vi "HW_set_IO_ports_3-pos_2.vi"(0 "IO parameters cluster":T1) -> (1 "IO parameters cluster output":T1, 2 "IO changed":bool)   [LabVIEW 2018, in "Tracker.lvlib"]
uses:
  Tracker.lvlib
  Controls/CTL_IO_params_cluster.ctl
  <vilib>/Utility/miscctls.llb/LVPointTypeDef.ctl
panel:
  out "In tag":string
  out "Out tag":string
  in  "IO 4 invert":bool caption="Swap High/Low"
  in  "IO 3 invert":bool caption="Swap High/Low"
  in  "IO 2 invert":bool caption="Swap High/Low"
  in  "IO 1 invert":bool caption="Swap High/Low"
  in  "IO 4":u16(ring)=1 items=["Out", "In"]
  in  "IO 3":u16(ring)=1 items=["Out", "In"]
  in  "IO 2":u16(ring) items=["Out", "In", "Sync (p)"]
  in  "IO 1":u16(ring) items=["Out", "In", "Sync (t)"]
  in  "Activate ext. RS-232":bool
  in  "Reset IO":bool
  in  "IO 4 start/stop":bool caption="Send TTL at Start and Stop"
  in  "IO 3 start/stop":bool caption="Send TTL at Start and Stop"
  in  "IO 2 start/stop":bool caption="Initiate outgoing TTL pulse"
  in  "IO 1 start/stop":bool caption="Initiate outgoing TTL pulse"
  in  "Exit":bool
  in  "Save Settings":bool
  in  "IO 4 zone":bool
  in  "IO 3 zone":bool
  in  "IO 2 sync":bool
  in  "IO 2 zone":bool=TRUE
  in  "IO 1 sync":bool
  in  "IO 1 zone":bool=TRUE
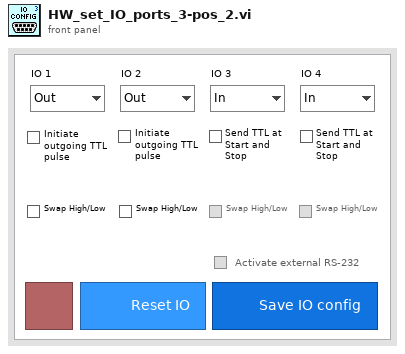
[diagram p1: front panel]
types:
  T1 = typedef "Tracker.lvlib/CTL_IO_params_cluster.ctl" = cluster{"IO general config.":u16, "IO 1 configuration":u16, "IO 2 configuration":u16, "IO 3 configuration":u16, "IO 4 configuration":u16, "Activate ext. RS-232":u16, "IO inversion config.":u16, "Sync capability":u8}
  T2 = typedef "LVPointTypeDef.ctl" = cluster{"Horizontal":i16, "Vertical":i16}
  T3 = enum8{"Enabled", "Disabled", "Disabled and Grayed Out"}
  T4 = cluster{"IO general config.":bool, "IO 1 configuration":bool, "IO 2 configuration":bool, "IO 3 configuration":bool, "IO 4 configuration":bool, "Activate ext. RS-232":bool, "IO inversion config.":bool, "Sync capability":bool}
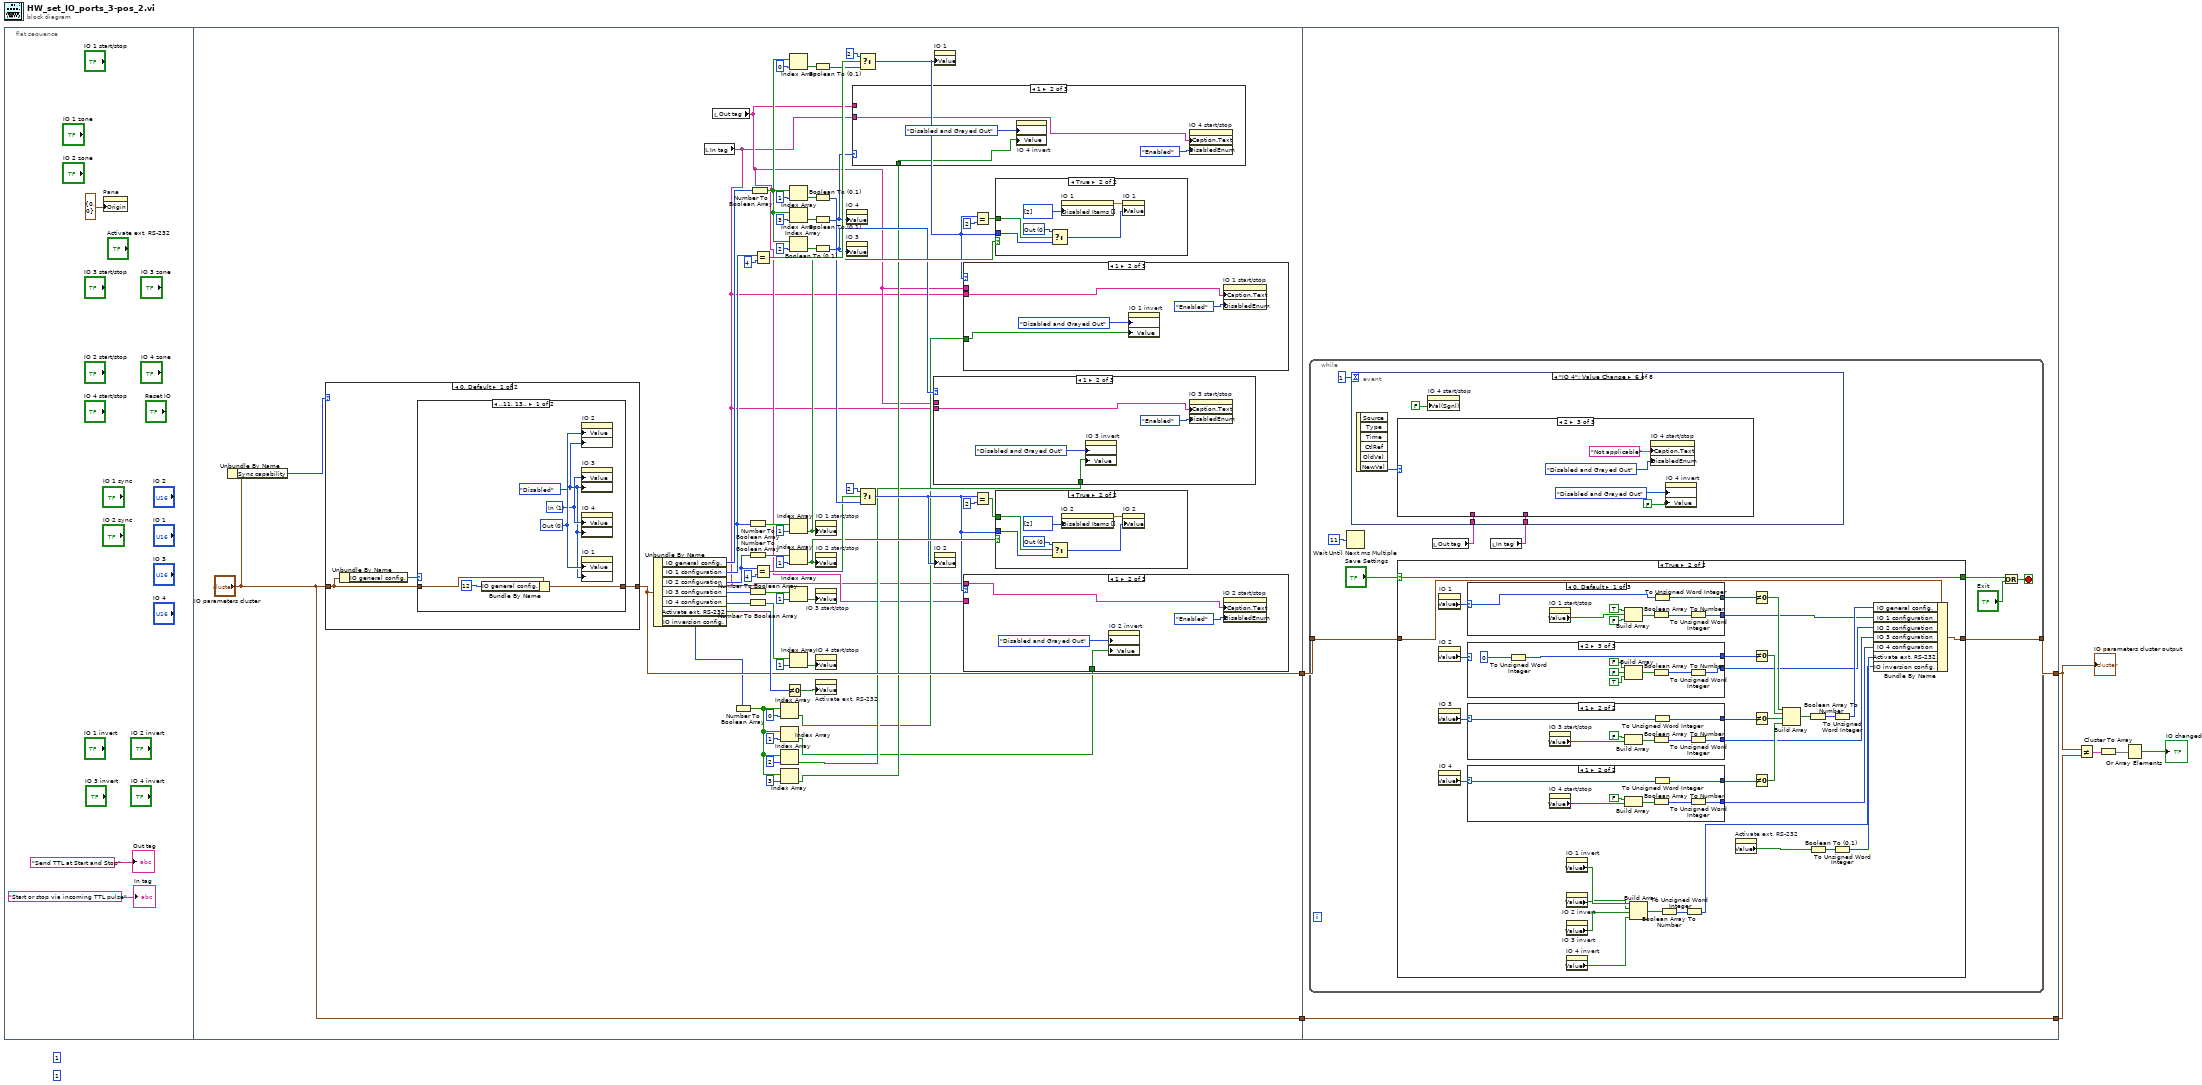
[diagram p0: block diagram]
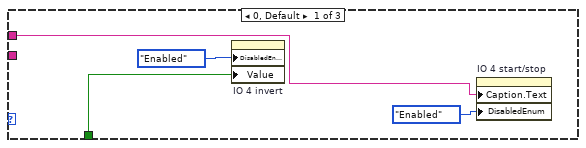
[diagram p2: hidden frame]
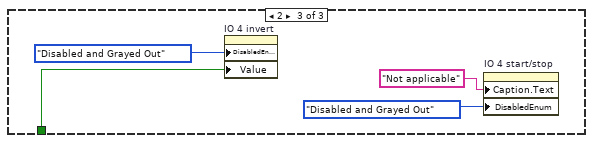
[diagram p3: hidden frame]
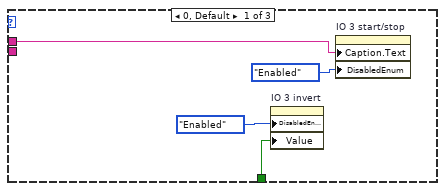
[diagram p4: hidden frame]
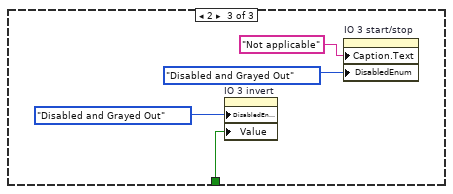
[diagram p5: hidden frame]
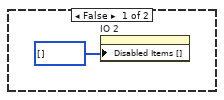
[diagram p6: hidden frame]
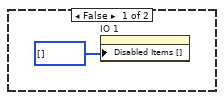
[diagram p7: hidden frame]
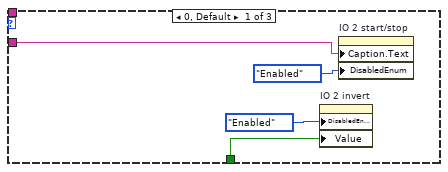
[diagram p8: hidden frame]
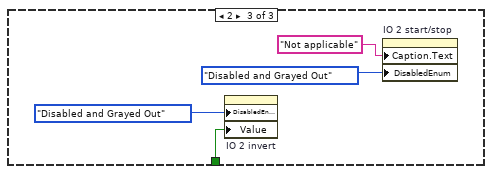
[diagram p9: hidden frame]
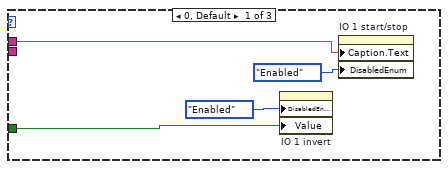
[diagram p10: hidden frame]
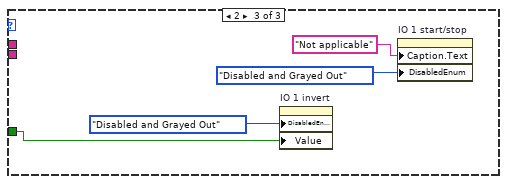
[diagram p11: hidden frame]
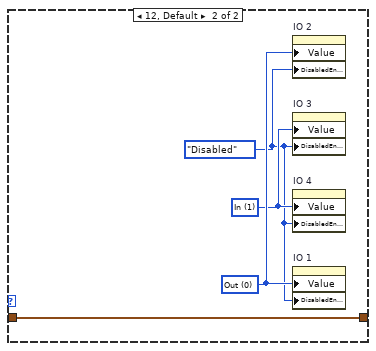
[diagram p12: hidden frame]
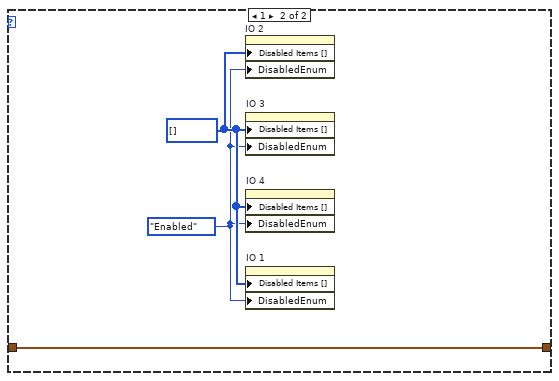
[diagram p13: hidden frame]
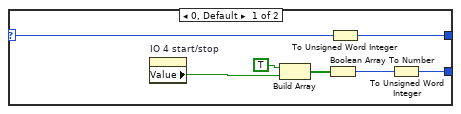
[diagram p15: hidden frame]
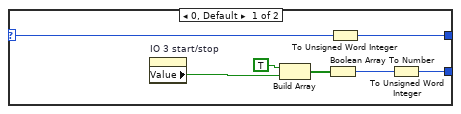
[diagram p16: hidden frame]
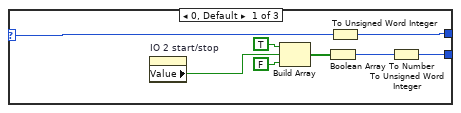
[diagram p17: hidden frame]
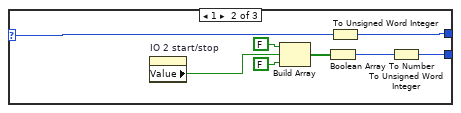
[diagram p18: hidden frame]
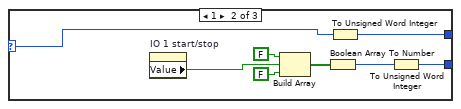
[diagram p19: hidden frame]
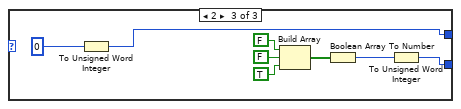
[diagram p20: hidden frame]
diagram:
  (unwired) 1 ("index")
  (unwired) 1 ("index")
  n1 = flat-sequence {
    tunnel: [w49] -> w7
    tunnel: ["IO parameters cluster"] -> w6
    tunnel: [w150] -> w5
    tunnel: w7 -> [w149]
    tunnel: w6 -> [w148]
    tunnel: [w148] -> w4
    frame #0 {
      n2 = property on="Pane" class="Pane"("Origin"=T2 {"Horizontal"=0, "Vertical"=0}) -> ()  [unwired: 2 in, 2 out]
      "In tag" <- "Start or stop via incoming TTL pulse" ("In tag")
      "Out tag" <- "Send TTL at Start and Stop" ("Out tag")
    }
    frame #1 {
      n3 = Unbundle By Name("IO parameters cluster") -> ("Sync capability"=w14:u8)
      n4 = case shown="0, Default" w14 {
        tunnel: "IO parameters cluster" -> [w133 w147]
        tunnel: [w132 w147] -> w49
        frame 0, Default {
          n5 = Unbundle By Name(w133) -> ("IO general config."=w134:u16)
          n6 = case shown="..11, 13.." w134 {
            tunnel: [w139 w144] -> w132
            tunnel: w133 -> [w140 w144]
            frame ..11, 13.. {
              w135 = T3."Disabled" ("Disabled")
              w136 = u16 1 items=["Out", "In"] ("IO 3")
              w137 = u16 0 items=["Out", "In", "Sync (t)"] ("IO 1")
              n7 = Bundle By Name(cluster=w140, "IO general config."=u16 12 ("SYNC configuration")) -> (w139:T1)
              n8 = property on="IO 2" class="Ring (strict)"("Value"=w137, "DisabledEnum"=w135) -> ()  [unwired: 2 in, 2 out]
              n9 = property on="IO 3" class="Ring (strict)"("Value"=w136, "DisabledEnum"=w135) -> ()  [unwired: 2 in, 2 out]
              n10 = property on="IO 4" class="Ring (strict)"("Value"=w136, "DisabledEnum"=w135) -> ()  [unwired: 2 in, 2 out]
              n11 = property on="IO 1" class="Ring (strict)"("Value"=w137, "DisabledEnum"=w135) -> ()  [unwired: 2 in, 2 out]
            }
            frame 12, Default {
              w141 = T3."Disabled" ("Disabled")
              w142 = u16 1 items=["Out", "In"] ("IO 3")
              w143 = u16 0 items=["Out", "In", "Sync (t)"] ("IO 1")
              n12 = property on="IO 2" class="Ring (strict)"("Value"=w143, "DisabledEnum"=w141) -> ()  [unwired: 2 in, 2 out]
              n13 = property on="IO 3" class="Ring (strict)"("Value"=w142, "DisabledEnum"=w141) -> ()  [unwired: 2 in, 2 out]
              n14 = property on="IO 4" class="Ring (strict)"("Value"=w142, "DisabledEnum"=w141) -> ()  [unwired: 2 in, 2 out]
              n15 = property on="IO 1" class="Ring (strict)"("Value"=w143, "DisabledEnum"=w141) -> ()  [unwired: 2 in, 2 out]
            }
          }
        }
        frame 1 {
          w145 = T3."Enabled" ("Disabled")
          w146 = i32[] [] ("Disabled Items []")
          n16 = property on="IO 2" class="Ring (strict)"("Disabled Items []"=w146, "DisabledEnum"=w145) -> ()  [unwired: 2 in, 2 out]
          n17 = property on="IO 3" class="Ring (strict)"("Disabled Items []"=w146, "DisabledEnum"=w145) -> ()  [unwired: 2 in, 2 out]
          n18 = property on="IO 4" class="Ring (strict)"("Disabled Items []"=w146, "DisabledEnum"=w145) -> ()  [unwired: 2 in, 2 out]
          n19 = property on="IO 1" class="Ring (strict)"("Disabled Items []"=w146, "DisabledEnum"=w145) -> ()  [unwired: 2 in, 2 out]
        }
      }
      n20 = Unbundle By Name(w49) -> ("IO general config."=w69:u16, "IO 1 configuration"=w44:u16, "IO 2 configuration"=w36:u16, "IO 3 configuration"=w53:u16, "IO 4 configuration"=w52:u16, "Activate ext. RS-232"=w51:u16, "IO inversion config."=w24:u16)
      n21 = local read "In tag"() -> (w11:string)
      n22 = local read "Out tag"() -> (w12:string)
      n23 = Number To Boolean Array(number=w24) -> (Boolean array=w19:bool[])
      n24 = Number To Boolean Array(number=w44) -> (Boolean array=w59:bool[])
      n25 = Number To Boolean Array(number=w36) -> (Boolean array=w56:bool[])
      n26 = Number To Boolean Array(number=w53) -> (Boolean array=w55:bool[])
      n27 = Number To Boolean Array(number=w52) -> (Boolean array=w45:bool[])
      n28 = Number To Boolean Array(number=w69) -> (Boolean array=w68:bool[])
      n29 = Equal?(x=w44, y=u16 4) -> (x = y?=w42:bool)
      n30 = Equal?(x=w36, y=u16 4) -> (x = y?=w35:bool)
      n31 = Index Array(array=w19, index=0) -> (element=w15:bool)
      n32 = Index Array(array=w19, index=1) -> (element=w16:bool)
      n33 = Index Array(array=w19, index=2) -> (element=w17:bool)
      n34 = Index Array(array=w19, index=3) -> (element=w18:bool)
      n35 = Not Equal To 0?(x=w51) -> (x != 0?=w50:bool)
      n36 = Index Array(array=w68, index=0) -> (element=w63:bool)
      n37 = Index Array(array=w68, index=1) -> (element=w62:bool)
      n38 = Index Array(array=w68, index=3) -> (element=w60:bool)
      n39 = Index Array(array=w68, index=2) -> (element=w61:bool)
      n40 = Index Array(array=w59, index=1) -> (element=w33:bool)
      n41 = Index Array(array=w56, index=1) -> (element=w28:bool)
      n42 = Index Array(array=w55, index=1) -> (element=w54:bool)
      n43 = Index Array(array=w45, index=1) -> (element=w46:bool)
      n44 = Boolean To (0,1)(Boolean=w63) -> (0, 1=w41:i16)
      n45 = Boolean To (0,1)(Boolean=w62) -> (0, 1=w38:i16)
      n46 = Boolean To (0,1)(Boolean=w60) -> (0, 1=w25:i16)
      n47 = Boolean To (0,1)(Boolean=w61) -> (0, 1=w26:i16)
      n48 = property on="IO 1 start/stop" class="Bool (strict)"("Value"=w33) -> ()  [unwired: 2 in, 2 out]
      n49 = property on="IO 2 start/stop" class="Bool (strict)"("Value"=w28) -> ()  [unwired: 2 in, 2 out]
      n50 = property on="IO 3 start/stop" class="Bool (strict)"("Value"=w54) -> ()  [unwired: 2 in, 2 out]
      n51 = property on="IO 4 start/stop" class="Bool (strict)"("Value"=w46) -> ()  [unwired: 2 in, 2 out]
      n52 = property on="Activate ext. RS-232" class="Bool (strict)"("Value"=w50) -> ()  [unwired: 2 in, 2 out]
      n53 = property on="IO 4" class="Ring (strict)"("Value"=w25) -> ()  [unwired: 2 in, 2 out]
      n54 = property on="IO 3" class="Ring (strict)"("Value"=w26) -> ()  [unwired: 2 in, 2 out]
      n55 = case shown="1" w25 {
        tunnel: w18 -> [w71 w75 w78]
        tunnel: w12 -> [w70 _ _]
        tunnel: w11 -> [_ w74 _]
        frame 0, Default {
          n56 = property on="IO 4 invert" class="Bool (strict)"("DisabledEnum"=T3."Enabled" ("Disabled"), "Value"=w71) -> ()  [unwired: 2 in, 2 out]
          n57 = property on="IO 4 start/stop" class="Bool (strict)"("Caption.Text"=w70, "DisabledEnum"=T3."Enabled" ("Disabled")) -> ()  [unwired: 2 in, 2 out]
        }
        frame 1 {
          n58 = property on="IO 4 invert" class="Bool (strict)"("DisabledEnum"=T3."Disabled and Grayed Out" ("Disabled"), "Value"=w75) -> ()  [unwired: 2 in, 2 out]
          n59 = property on="IO 4 start/stop" class="Bool (strict)"("Caption.Text"=w74, "DisabledEnum"=T3."Enabled" ("Disabled")) -> ()  [unwired: 2 in, 2 out]
        }
        frame 2 {
          n60 = property on="IO 4 invert" class="Bool (strict)"("DisabledEnum"=T3."Disabled and Grayed Out" ("Disabled"), "Value"=w78) -> ()  [unwired: 2 in, 2 out]
          n61 = property on="IO 4 start/stop" class="Bool (strict)"("Caption.Text"="Not applicable", "DisabledEnum"=T3."Disabled and Grayed Out" ("Disabled")) -> ()  [unwired: 2 in, 2 out]
        }
      }
      n62 = Select(t=i16 2, s=w42, f=w41) -> (s? t:f=w31:i16)
      n63 = Select(t=i16 2, s=w35, f=w38) -> (s? t:f=w27:i16)
      n64 = case shown="1" w26 {
        tunnel: w17 -> [w83 w87 w90]
        tunnel: w12 -> [w82 _ _]
        tunnel: w11 -> [_ w86 _]
        frame 0, Default {
          n65 = property on="IO 3 invert" class="Bool (strict)"("DisabledEnum"=T3."Enabled" ("Disabled"), "Value"=w83) -> ()  [unwired: 2 in, 2 out]
          n66 = property on="IO 3 start/stop" class="Bool (strict)"("Caption.Text"=w82, "DisabledEnum"=T3."Enabled" ("Disabled")) -> ()  [unwired: 2 in, 2 out]
        }
        frame 1 {
          n67 = property on="IO 3 invert" class="Bool (strict)"("DisabledEnum"=T3."Disabled and Grayed Out" ("Disabled"), "Value"=w87) -> ()  [unwired: 2 in, 2 out]
          n68 = property on="IO 3 start/stop" class="Bool (strict)"("Caption.Text"=w86, "DisabledEnum"=T3."Enabled" ("Disabled")) -> ()  [unwired: 2 in, 2 out]
        }
        frame 2 {
          n69 = property on="IO 3 invert" class="Bool (strict)"("DisabledEnum"=T3."Disabled and Grayed Out" ("Disabled"), "Value"=w90) -> ()  [unwired: 2 in, 2 out]
          n70 = property on="IO 3 start/stop" class="Bool (strict)"("Caption.Text"="Not applicable", "DisabledEnum"=T3."Disabled and Grayed Out" ("Disabled")) -> ()  [unwired: 2 in, 2 out]
        }
      }
      n71 = property on="IO 1" class="Ring (strict)"("Value"=w31) -> ()  [unwired: 2 in, 2 out]
      n72 = property on="IO 2" class="Ring (strict)"("Value"=w27) -> ()  [unwired: 2 in, 2 out]
      n73 = case shown="1" w31 {
        tunnel: w15 -> [w121 w125 w128]
        tunnel: w12 -> [w120 _ _]
        tunnel: w11 -> [_ w124 _]
        frame 0, Default {
          n74 = property on="IO 1 invert" class="Bool (strict)"("DisabledEnum"=T3."Enabled" ("Disabled"), "Value"=w121) -> ()  [unwired: 2 in, 2 out]
          n75 = property on="IO 1 start/stop" class="Bool (strict)"("Caption.Text"=w120, "DisabledEnum"=T3."Enabled" ("Disabled")) -> ()  [unwired: 2 in, 2 out]
        }
        frame 1 {
          n76 = property on="IO 1 invert" class="Bool (strict)"("DisabledEnum"=T3."Disabled and Grayed Out" ("Disabled"), "Value"=w125) -> ()  [unwired: 2 in, 2 out]
          n77 = property on="IO 1 start/stop" class="Bool (strict)"("Caption.Text"=w124, "DisabledEnum"=T3."Enabled" ("Disabled")) -> ()  [unwired: 2 in, 2 out]
        }
        frame 2 {
          n78 = property on="IO 1 invert" class="Bool (strict)"("DisabledEnum"=T3."Disabled and Grayed Out" ("Disabled"), "Value"=w128) -> ()  [unwired: 2 in, 2 out]
          n79 = property on="IO 1 start/stop" class="Bool (strict)"("Caption.Text"="Not applicable", "DisabledEnum"=T3."Disabled and Grayed Out" ("Disabled")) -> ()  [unwired: 2 in, 2 out]
        }
      }
      n80 = case shown="1" w27 {
        tunnel: w16 -> [w109 w113 w116]
        tunnel: w12 -> [w108 _ _]
        tunnel: w11 -> [_ w112 _]
        frame 0, Default {
          n81 = property on="IO 2 invert" class="Bool (strict)"("DisabledEnum"=T3."Enabled" ("Disabled"), "Value"=w109) -> ()  [unwired: 2 in, 2 out]
          n82 = property on="IO 2 start/stop" class="Bool (strict)"("Caption.Text"=w108, "DisabledEnum"=T3."Enabled" ("Disabled")) -> ()  [unwired: 2 in, 2 out]
        }
        frame 1 {
          n83 = property on="IO 2 invert" class="Bool (strict)"("DisabledEnum"=T3."Disabled and Grayed Out" ("Disabled"), "Value"=w113) -> ()  [unwired: 2 in, 2 out]
          n84 = property on="IO 2 start/stop" class="Bool (strict)"("Caption.Text"=w112, "DisabledEnum"=T3."Enabled" ("Disabled")) -> ()  [unwired: 2 in, 2 out]
        }
        frame 2 {
          n85 = property on="IO 2 invert" class="Bool (strict)"("DisabledEnum"=T3."Disabled and Grayed Out" ("Disabled"), "Value"=w116) -> ()  [unwired: 2 in, 2 out]
          n86 = property on="IO 2 start/stop" class="Bool (strict)"("Caption.Text"="Not applicable", "DisabledEnum"=T3."Disabled and Grayed Out" ("Disabled")) -> ()  [unwired: 2 in, 2 out]
        }
      }
      n87 = Equal?(x=w31, y=u16 2) -> (x = y?=w34:bool)
      n88 = Equal?(x=w27, y=u16 2) -> (x = y?=w30:bool)
      n89 = case shown="True" w33 {
        tunnel: w34 -> [_ w105]
        tunnel: w31 -> [_ w102]
        frame False {
          n90 = property on="IO 1" class="Ring (strict)"("Disabled Items []"=i32[] []) -> ()  [unwired: 2 in, 2 out]
        }
        frame True {
          w104 = u16 0 items=["Out", "In", "Sync (t)"] ("IO 1")
          n91 = Select(t=w104, s=w105, f=w102) -> (s? t:f=w103:u16)
          n92 = property on="IO 1" class="Ring (strict)"("Disabled Items []"=i32[] [2]) -> (error out=w106:errorcluster)  [unwired: 2 in, 1 out]
          n93 = property on="IO 1" class="Ring (strict)"(error in=w106, "Value"=w103) -> ()  [unwired: 1 in, 2 out]
        }
      }
      n94 = case shown="True" w28 {
        tunnel: w30 -> [_ w98]
        tunnel: w27 -> [_ w95]
        frame False {
          n95 = property on="IO 2" class="Ring (strict)"("Disabled Items []"=i32[] []) -> ()  [unwired: 2 in, 2 out]
        }
        frame True {
          w97 = u16 0 items=["Out", "In", "Sync (t)"] ("IO 1")
          n96 = Select(t=w97, s=w98, f=w95) -> (s? t:f=w96:u16)
          n97 = property on="IO 2" class="Ring (strict)"("Disabled Items []"=i32[] [2]) -> (error out=w99:errorcluster)  [unwired: 2 in, 1 out]
          n98 = property on="IO 2" class="Ring (strict)"(error in=w99, "Value"=w96) -> ()  [unwired: 1 in, 2 out]
        }
      }
    }
    frame #2 {
      n99 = while {
        tunnel: [w154] -> w150
        tunnel: w149 -> [w153]
        stop <- w157 stop-if-true
        n100 = Wait Until Next ms Multiple(millisecond multiple=u32 11) -> ()  [unwired: 1 out]
        n101 = case shown="True" "Save Settings" {
          selector: "Save Settings" -> [w162 w194]
          tunnel: [w162 w194] -> w155
          tunnel: [w161 w189] -> w154
          tunnel: w153 -> [w161 w190]
          frame False {
          }
          frame True {
            n102 = property on="IO 1" class="Ring (strict)"() -> ("Value"=w191:u16)  [unwired: 2 in, 2 out]
            n103 = property on="IO 2" class="Ring (strict)"() -> ("Value"=w188:u16)  [unwired: 2 in, 2 out]
            n104 = property on="IO 3" class="Ring (strict)"() -> ("Value"=w187:u16)  [unwired: 2 in, 2 out]
            n105 = property on="IO 4" class="Ring (strict)"() -> ("Value"=w186:u16)  [unwired: 2 in, 2 out]
            n106 = case shown="0, Default" w191 {
              selector: w191 -> [w250 w258 _]
              tunnel: [w247 w255 w264] -> w174
              tunnel: [w249 w257 w267] -> w179
              frame 0, Default {
                n107 = property on="IO 1 start/stop" class="Bool (strict)"() -> ("Value"=w254:bool)  [unwired: 2 in, 2 out]
                n108 = Build Array(TRUE, w254, FALSE) -> (w251:bool[])
                n109 = Boolean Array To Number(Boolean array=w251) -> (number=w248:u32)
                n110 = To Unsigned Word Integer(number=w250) -> (unsigned 16bit integer=w249:u16)
                n111 = To Unsigned Word Integer(number=w248) -> (unsigned 16bit integer=w247:u16)
              }
              frame 1 {
                n112 = property on="IO 1 start/stop" class="Bool (strict)"() -> ("Value"=w262:bool)  [unwired: 2 in, 2 out]
                n113 = Build Array(FALSE, w262, FALSE) -> (w259:bool[])
                n114 = Boolean Array To Number(Boolean array=w259) -> (number=w256:u32)
                n115 = To Unsigned Word Integer(number=w258) -> (unsigned 16bit integer=w257:u16)
                n116 = To Unsigned Word Integer(number=w256) -> (unsigned 16bit integer=w255:u16)
              }
              frame 2 {
                n117 = To Unsigned Word Integer(number=u16 0) -> (unsigned 16bit integer=w267:u16)
                n118 = Build Array(FALSE, FALSE, TRUE) -> (w268:bool[])
                n119 = Boolean Array To Number(Boolean array=w268) -> (number=w265:u32)
                n120 = To Unsigned Word Integer(number=w265) -> (unsigned 16bit integer=w264:u16)
              }
            }
            n121 = case shown="2" w188 {
              selector: w188 -> [w226 w234 _]
              tunnel: [w223 w231 w240] -> w173
              tunnel: [w225 w233 w243] -> w178
              frame 0, Default {
                n122 = property on="IO 2 start/stop" class="Bool (strict)"() -> ("Value"=w230:bool)  [unwired: 2 in, 2 out]
                n123 = Build Array(TRUE, w230, FALSE) -> (w227:bool[])
                n124 = Boolean Array To Number(Boolean array=w227) -> (number=w224:u32)
                n125 = To Unsigned Word Integer(number=w226) -> (unsigned 16bit integer=w225:u16)
                n126 = To Unsigned Word Integer(number=w224) -> (unsigned 16bit integer=w223:u16)
              }
              frame 1 {
                n127 = property on="IO 2 start/stop" class="Bool (strict)"() -> ("Value"=w238:bool)  [unwired: 2 in, 2 out]
                n128 = Build Array(FALSE, w238, FALSE) -> (w235:bool[])
                n129 = Boolean Array To Number(Boolean array=w235) -> (number=w232:u32)
                n130 = To Unsigned Word Integer(number=w234) -> (unsigned 16bit integer=w233:u16)
                n131 = To Unsigned Word Integer(number=w232) -> (unsigned 16bit integer=w231:u16)
              }
              frame 2 {
                n132 = To Unsigned Word Integer(number=u16 0) -> (unsigned 16bit integer=w243:u16)
                n133 = Build Array(FALSE, FALSE, TRUE) -> (w244:bool[])
                n134 = Boolean Array To Number(Boolean array=w244) -> (number=w241:u32)
                n135 = To Unsigned Word Integer(number=w241) -> (unsigned 16bit integer=w240:u16)
              }
            }
            n136 = case shown="1" w187 {
              selector: w187 -> [w212 w219]
              tunnel: [w209 w216] -> w172
              tunnel: [w211 w218] -> w177
              frame 0, Default {
                n137 = property on="IO 3 start/stop" class="Bool (strict)"() -> ("Value"=w215:bool)  [unwired: 2 in, 2 out]
                n138 = Build Array(TRUE, w215) -> (w213:bool[])
                n139 = Boolean Array To Number(Boolean array=w213) -> (number=w210:u32)
                n140 = To Unsigned Word Integer(number=w212) -> (unsigned 16bit integer=w211:u16)
                n141 = To Unsigned Word Integer(number=w210) -> (unsigned 16bit integer=w209:u16)
              }
              frame 1 {
                n142 = property on="IO 3 start/stop" class="Bool (strict)"() -> ("Value"=w222:bool)  [unwired: 2 in, 2 out]
                n143 = Build Array(FALSE, w222) -> (w220:bool[])
                n144 = Boolean Array To Number(Boolean array=w220) -> (number=w217:u32)
                n145 = To Unsigned Word Integer(number=w219) -> (unsigned 16bit integer=w218:u16)
                n146 = To Unsigned Word Integer(number=w217) -> (unsigned 16bit integer=w216:u16)
              }
            }
            n147 = case shown="1" w186 {
              selector: w186 -> [w198 w205]
              tunnel: [w195 w202] -> w171
              tunnel: [w197 w204] -> w176
              frame 0, Default {
                n148 = property on="IO 4 start/stop" class="Bool (strict)"() -> ("Value"=w201:bool)  [unwired: 2 in, 2 out]
                n149 = Build Array(TRUE, w201) -> (w199:bool[])
                n150 = Boolean Array To Number(Boolean array=w199) -> (number=w196:u32)
                n151 = To Unsigned Word Integer(number=w198) -> (unsigned 16bit integer=w197:u16)
                n152 = To Unsigned Word Integer(number=w196) -> (unsigned 16bit integer=w195:u16)
              }
              frame 1 {
                n153 = property on="IO 4 start/stop" class="Bool (strict)"() -> ("Value"=w208:bool)  [unwired: 2 in, 2 out]
                n154 = Build Array(FALSE, w208) -> (w206:bool[])
                n155 = Boolean Array To Number(Boolean array=w206) -> (number=w203:u32)
                n156 = To Unsigned Word Integer(number=w205) -> (unsigned 16bit integer=w204:u16)
                n157 = To Unsigned Word Integer(number=w203) -> (unsigned 16bit integer=w202:u16)
              }
            }
            n158 = property on="IO 1 invert" class="Bool (strict)"() -> ("Value"=w169:bool)  [unwired: 2 in, 2 out]
            n159 = property on="IO 2 invert" class="Bool (strict)"() -> ("Value"=w168:bool)  [unwired: 2 in, 2 out]
            n160 = property on="IO 3 invert" class="Bool (strict)"() -> ("Value"=w167:bool)  [unwired: 2 in, 2 out]
            n161 = property on="IO 4 invert" class="Bool (strict)"() -> ("Value"=w166:bool)  [unwired: 2 in, 2 out]
            n162 = Build Array(w169, w168, w167, w166) -> (w164:bool[])
            n163 = Boolean Array To Number(Boolean array=w164) -> (number=w165:u32)
            n164 = To Unsigned Word Integer(number=w165) -> (unsigned 16bit integer=w163:u16)
            n165 = property on="Activate ext. RS-232" class="Bool (strict)"() -> ("Value"=w193:bool)  [unwired: 2 in, 2 out]
            n166 = Not Equal To 0?(x=w179) -> (x != 0?=w185:bool)
            n167 = Not Equal To 0?(x=w178) -> (x != 0?=w184:bool)
            n168 = Not Equal To 0?(x=w177) -> (x != 0?=w183:bool)
            n169 = Not Equal To 0?(x=w176) -> (x != 0?=w182:bool)
            n170 = Build Array(w185, w184, w183, w182) -> (w181:bool[])
            n171 = Boolean Array To Number(Boolean array=w181) -> (number=w180:u32)
            n172 = Boolean To (0,1)(Boolean=w193) -> (0, 1=w192:i16)
            n173 = To Unsigned Word Integer(number=w180) -> (unsigned 16bit integer=w175:u16)
            n174 = To Unsigned Word Integer(number=w192) -> (unsigned 16bit integer=w170:u16)
            n175 = Bundle By Name(cluster=w190, "IO general config."=w175, "IO 1 configuration"=w174, "IO 2 configuration"=w173, "IO 3 configuration"=w172, "IO 4 configuration"=w171, "Activate ext. RS-232"=w170, "IO inversion config."=w163) -> (w189:T1)
          }
        }
        n176 = local read "Out tag"() -> (w152:string)
        n177 = local read "In tag"() -> (w151:string)
        n178 = event shown="[5] \"IO 4\": Value Change" {
          selector: _ -> [_ _ _ _ _ _ _ _]
          dyn-events: _ -> [_ _ _ _ _ _ _ _]
          timeout: 1 -> [_ _ _ _ _ _ _ _]
          tunnel: w152 -> [_ _ w294 w307 w321 w335 _ _]
          tunnel: w151 -> [_ _ w293 w306 w320 w334 _ _]
          event Timeout {
            n179 = event-data() -> ()  [unwired: 1 in, 3 out]
          }
          event "Reset IO": Value Change {
            w282 = u16 1 ("Value (Signaling)")
            w283 = u16 0 ("Value (Signaling)")
            w277 = FALSE ("Value (Signaling)")
            n180 = event-data() -> ()  [unwired: 1 in, 6 out]
            n181 = property on="IO 1" class="Ring (strict)"("Val(Sgnl)"=w283) -> (error out=w281:errorcluster)  [unwired: 2 in, 1 out]
            n182 = property on="IO 2" class="Ring (strict)"("Val(Sgnl)"=w283) -> (error out=w280:errorcluster)  [unwired: 2 in, 1 out]
            n183 = property on="IO 3" class="Ring (strict)"("Val(Sgnl)"=w282) -> (error out=w290:errorcluster)  [unwired: 2 in, 1 out]
            n184 = property on="IO 4" class="Ring (strict)"("Val(Sgnl)"=w282) -> (error out=w288:errorcluster)  [unwired: 2 in, 1 out]
            n185 = property on="IO 1 start/stop" class="Bool (strict)"(error in=w281, "Val(Sgnl)"=w277) -> (error out=w279:errorcluster)  [unwired: 1 in, 1 out]
            n186 = property on="IO 2 start/stop" class="Bool (strict)"(error in=w280, "Val(Sgnl)"=FALSE ("Value (Signaling)")) -> (error out=w276:errorcluster)  [unwired: 1 in, 1 out]
            n187 = property on="IO 3 start/stop" class="Bool (strict)"(error in=w290, "Val(Sgnl)"=FALSE ("Value (Signaling)")) -> (error out=w275:errorcluster)  [unwired: 1 in, 1 out]
            n188 = property on="IO 4 start/stop" class="Bool (strict)"(error in=w288, "Val(Sgnl)"=FALSE ("Value (Signaling)")) -> (error out=w274:errorcluster)  [unwired: 1 in, 1 out]
            n189 = property on="IO 1 invert" class="Bool (strict)"(error in=w279, "Val(Sgnl)"=w277) -> (error out=w278:errorcluster)  [unwired: 1 in, 1 out]
            n190 = property on="IO 2 invert" class="Bool (strict)"(error in=w276, "Val(Sgnl)"=w277) -> (error out=w273:errorcluster)  [unwired: 1 in, 1 out]
            n191 = property on="IO 3 invert" class="Bool (strict)"(error in=w275, "Val(Sgnl)"=w277) -> (error out=w272:errorcluster)  [unwired: 1 in, 1 out]
            n192 = property on="IO 4 invert" class="Bool (strict)"(error in=w274, "Val(Sgnl)"=w277) -> (error out=w271:errorcluster)  [unwired: 1 in, 1 out]
            n193 = Merge Errors(w278, w273, w272, w271) -> (w287:errorcluster)
            n194 = property on="Reset IO" class="Bool (strict)"(error in=w287, "Value"=FALSE ("Reset IO")) -> (error out=w284:errorcluster)  [unwired: 1 in, 1 out]
            n195 = property on="Activate ext. RS-232" class="Bool (strict)"(error in=w284, "Value"=FALSE ("Activate ext. RS-232")) -> ()  [unwired: 1 in, 2 out]
          }
          event "IO 1": Value Change {
            n196 = event-data() -> ("NewVal"=w295:u16)  [unwired: 1 in, 5 out]
            n197 = case shown="2" w295 {
              tunnel: w294 -> [w297 _ _]
              tunnel: w293 -> [_ w299 _]
              frame 0, Default {
                w298 = T3."Enabled" ("Disabled")
                n198 = property on="IO 1 start/stop" class="Bool (strict)"("Caption.Text"=w297, "DisabledEnum"=w298) -> ()  [unwired: 2 in, 2 out]
                n199 = property on="IO 1 invert" class="Bool (strict)"("DisabledEnum"=w298) -> ()  [unwired: 2 in, 2 out]
              }
              frame 1 {
                n200 = property on="IO 1 invert" class="Bool (strict)"("DisabledEnum"=T3."Disabled and Grayed Out" ("Disabled"), "Value"=FALSE ("IO 1 invert")) -> ()  [unwired: 2 in, 2 out]
                n201 = property on="IO 1 start/stop" class="Bool (strict)"("Caption.Text"=w299, "DisabledEnum"=T3."Enabled" ("Disabled")) -> ()  [unwired: 2 in, 2 out]
              }
              frame 2 {
                w304 = T3."Disabled and Grayed Out" ("Disabled")
                n202 = property on="IO 1 start/stop" class="Bool (strict)"("Caption.Text"="Not applicable", "DisabledEnum"=w304) -> ()  [unwired: 2 in, 2 out]
                n203 = property on="IO 1 invert" class="Bool (strict)"("DisabledEnum"=w304, "Value"=FALSE ("IO 1 invert")) -> ()  [unwired: 2 in, 2 out]
              }
            }
            n204 = property on="IO 1 start/stop" class="Bool (strict)"("Val(Sgnl)"=FALSE ("IO 1 start/stop")) -> ()  [unwired: 2 in, 2 out]
          }
          event "IO 2": Value Change {
            n205 = event-data() -> ("NewVal"=w308:u16)  [unwired: 1 in, 5 out]
            n206 = case shown="2" w308 {
              tunnel: w307 -> [w310 _ _]
              tunnel: w306 -> [_ w312 _]
              frame 0, Default {
                w311 = T3."Enabled" ("Disabled")
                n207 = property on="IO 2 start/stop" class="Bool (strict)"("Caption.Text"=w310, "DisabledEnum"=w311) -> ()  [unwired: 2 in, 2 out]
                n208 = property on="IO 2 invert" class="Bool (strict)"("DisabledEnum"=w311) -> ()  [unwired: 2 in, 2 out]
              }
              frame 1 {
                n209 = property on="IO 2 start/stop" class="Bool (strict)"("Caption.Text"=w312, "DisabledEnum"=T3."Enabled" ("Disabled")) -> ()  [unwired: 2 in, 2 out]
                n210 = property on="IO 2 invert" class="Bool (strict)"("DisabledEnum"=T3."Disabled and Grayed Out" ("Disabled"), "Value"=FALSE ("IO 1 invert")) -> ()  [unwired: 2 in, 2 out]
              }
              frame 2 {
                n211 = property on="IO 2 start/stop" class="Bool (strict)"("Caption.Text"="Not applicable", "DisabledEnum"=T3."Disabled and Grayed Out" ("Disabled")) -> ()  [unwired: 2 in, 2 out]
                n212 = property on="IO 2 invert" class="Bool (strict)"("DisabledEnum"=T3."Disabled and Grayed Out" ("Disabled"), "Value"=FALSE ("IO 1 invert")) -> ()  [unwired: 2 in, 2 out]
              }
            }
            n213 = property on="IO 2 start/stop" class="Bool (strict)"("Val(Sgnl)"=FALSE ("IO 1 start/stop")) -> ()  [unwired: 2 in, 2 out]
          }
          event "IO 3": Value Change {
            n214 = event-data() -> ("NewVal"=w322:u16)  [unwired: 1 in, 5 out]
            n215 = case shown="2" w322 {
              tunnel: w321 -> [w324 _ _]
              tunnel: w320 -> [_ w326 _]
              frame 0, Default {
                w325 = T3."Enabled" ("Disabled")
                n216 = property on="IO 3 start/stop" class="Bool (strict)"("Caption.Text"=w324, "DisabledEnum"=w325) -> ()  [unwired: 2 in, 2 out]
                n217 = property on="IO 3 invert" class="Bool (strict)"("DisabledEnum"=w325) -> ()  [unwired: 2 in, 2 out]
              }
              frame 1 {
                n218 = property on="IO 3 start/stop" class="Bool (strict)"("Caption.Text"=w326, "DisabledEnum"=T3."Enabled" ("Disabled")) -> ()  [unwired: 2 in, 2 out]
                n219 = property on="IO 3 invert" class="Bool (strict)"("DisabledEnum"=T3."Disabled and Grayed Out" ("Disabled"), "Value"=FALSE ("IO 1 invert")) -> ()  [unwired: 2 in, 2 out]
              }
              frame 2 {
                n220 = property on="IO 3 start/stop" class="Bool (strict)"("Caption.Text"="Not applicable", "DisabledEnum"=T3."Disabled and Grayed Out" ("Disabled")) -> ()  [unwired: 2 in, 2 out]
                n221 = property on="IO 3 invert" class="Bool (strict)"("DisabledEnum"=T3."Disabled and Grayed Out" ("Disabled"), "Value"=FALSE ("IO 1 invert")) -> ()  [unwired: 2 in, 2 out]
              }
            }
            n222 = property on="IO 3 start/stop" class="Bool (strict)"("Val(Sgnl)"=FALSE ("IO 1 start/stop")) -> ()  [unwired: 2 in, 2 out]
          }
          event "IO 4": Value Change {
            n223 = event-data() -> ("NewVal"=w336:u16)  [unwired: 1 in, 5 out]
            n224 = case shown="2" w336 {
              tunnel: w335 -> [w338 _ _]
              tunnel: w334 -> [_ w340 _]
              frame 0, Default {
                w339 = T3."Enabled" ("Disabled")
                n225 = property on="IO 4 start/stop" class="Bool (strict)"("Caption.Text"=w338, "DisabledEnum"=w339) -> ()  [unwired: 2 in, 2 out]
                n226 = property on="IO 4 invert" class="Bool (strict)"("DisabledEnum"=w339) -> ()  [unwired: 2 in, 2 out]
              }
              frame 1 {
                n227 = property on="IO 4 start/stop" class="Bool (strict)"("Caption.Text"=w340, "DisabledEnum"=T3."Enabled" ("Disabled")) -> ()  [unwired: 2 in, 2 out]
                n228 = property on="IO 4 invert" class="Bool (strict)"("DisabledEnum"=T3."Disabled and Grayed Out" ("Disabled"), "Value"=FALSE ("IO 1 invert")) -> ()  [unwired: 2 in, 2 out]
              }
              frame 2 {
                n229 = property on="IO 4 start/stop" class="Bool (strict)"("Caption.Text"="Not applicable", "DisabledEnum"=T3."Disabled and Grayed Out" ("Disabled")) -> ()  [unwired: 2 in, 2 out]
                n230 = property on="IO 4 invert" class="Bool (strict)"("DisabledEnum"=T3."Disabled and Grayed Out" ("Disabled"), "Value"=FALSE ("IO 1 invert")) -> ()  [unwired: 2 in, 2 out]
              }
            }
            n231 = property on="IO 4 start/stop" class="Bool (strict)"("Val(Sgnl)"=FALSE ("IO 1 start/stop")) -> ()  [unwired: 2 in, 2 out]
          }
          event "IO 1 start/stop": Value Change {
            n232 = event-data() -> ("NewVal"=w349:bool)  [unwired: 1 in, 5 out]
            n233 = property on="IO 1" class="Ring (strict)"() -> ("Value"=w348:u16)  [unwired: 2 in, 2 out]
            n234 = Equal?(x=w348, y=u16 2) -> (x = y?=w350:bool)
            n235 = case shown="True" w349 {
              tunnel: w350 -> [_ w356]
              tunnel: w348 -> [_ w353]
              frame False {
                n236 = property on="IO 1" class="Ring (strict)"("Disabled Items []"=i32[] []) -> ()  [unwired: 2 in, 2 out]
              }
              frame True {
                w355 = u16 0 items=["Out", "In", "Sync (t)"] ("IO 1")
                n237 = Select(t=w355, s=w356, f=w353) -> (s? t:f=w354:u16)
                n238 = property on="IO 1" class="Ring (strict)"("Disabled Items []"=i32[] [2]) -> (error out=w357:errorcluster)  [unwired: 2 in, 1 out]
                n239 = property on="IO 1" class="Ring (strict)"(error in=w357, "Value"=w354) -> ()  [unwired: 1 in, 2 out]
              }
            }
          }
          event "IO 2 start/stop": Value Change {
            n240 = event-data() -> ("NewVal"=w360:bool)  [unwired: 1 in, 5 out]
            n241 = property on="IO 2" class="Ring (strict)"() -> ("Value"=w359:u16)  [unwired: 2 in, 2 out]
            n242 = Equal?(x=w359, y=u16 2) -> (x = y?=w361:bool)
            n243 = case shown="True" w360 {
              tunnel: w361 -> [_ w367]
              tunnel: w359 -> [_ w364]
              frame False {
                n244 = property on="IO 2" class="Ring (strict)"("Disabled Items []"=i32[] []) -> ()  [unwired: 2 in, 2 out]
              }
              frame True {
                w366 = u16 0 items=["Out", "In", "Sync (t)"] ("IO 1")
                n245 = Select(t=w366, s=w367, f=w364) -> (s? t:f=w365:u16)
                n246 = property on="IO 2" class="Ring (strict)"("Disabled Items []"=i32[] [2]) -> (error out=w368:errorcluster)  [unwired: 2 in, 1 out]
                n247 = property on="IO 2" class="Ring (strict)"(error in=w368, "Value"=w365) -> ()  [unwired: 1 in, 2 out]
              }
            }
          }
        }
        n248 = Or(x=w155, y="Exit") -> (x .or. y?=w157:bool)
      }
    }
  }
  n249 = Not Equal?(x=w5, y=w4) -> (x != y?=w3:T4)
  n250 = Cluster To Array(cluster=w3) -> (array=w2:bool[])
  n251 = Or Array Elements(Boolean array=w2) -> (logical OR=→"IO changed":bool)
  "IO parameters cluster output" <- w5
